vi "Actor Core.vi"(8 "error in":errorcluster, 11 "Nested in":refnum<class "Top Level.lvclass">) -> (0 "error out":errorcluster, 3 "Actor out":refnum<class "Actor.lvclass">)   [LabVIEW 2021, in "Top Level.lvlib" / "Top Level.lvclass"]
doc: "(<B>Filename</B>: Actor Framework.lvlib:Actor.lvclass:Actor Core.vi)\n\nReceives messages to the actor, reacts to them, and initiates any error handling that may shut the actor down.\n\nDescendant classes may override this VI to append parallel tasks for the actor to complete while it handles messages. Overrides use the Call Parent Method node."
uses:
  Top Level.lvclass
  C:/Program Files/National Instruments/LabVIEW 2021/vi.lib/ActorFramework/Actor/Actor.lvclass
  <vilib>/ActorFramework/Actor/Actor.lvclass
  <vilib>/ActorFramework/Actor/Actor.lvclass/Actor.ctl
  <vilib>/ActorFramework/Message Enqueuer/Message Enqueuer.lvclass/Message Enqueuer.ctl
  Top Level.lvclass/Top Level.ctl
  Top Level Messages/Password Authentication Msg/Password Authentication Msg.lvclass/Password Authentication Msg.ctl
  <vilib>/ActorFramework/Message Enqueuer/Init from Existing Queue.vi
  <vilib>/ActorFramework/Message Enqueuer/Enqueue.vi
  Top Level Messages/Password Authentication Msg/Password Authentication Msg.lvclass
  C:/Program Files/National Instruments/LabVIEW 2021/vi.lib/ActorFramework/Message/Message.lvclass
  <vilib>/ActorFramework/Stop Msg/Stop Msg.lvclass
  Top Level Messages/Reset Graph Msg/Reset Graph Msg.lvclass
  <vilib>/ActorFramework/Message Priority Queue/Priority Enqueue.vi
  <vilib>/ActorFramework/Message Enqueuer/Message Enqueuer.lvclass
  <vilib>/MGI/Panel Manager/Panel Actor/Panel Actor/Panel Actor.lvclass
panel:
  in  "Reset Graph":bool
  out "String":string="PH316 IV Curve Lab\n\nInstructions:\n\nCheck the user manual for hardware assembly.\n\nTo curve fit data to analytical functions, first export the necessary X-axis and Y-axis data:\nClick any of the three legends -> Export -> Export Data To ..\n\nCheck python's scipy.optimize.curve_fit module for details fitting your objective function to the data, further extracting unknown parameters of interest.\n\nZoom in / out, pane around, scale regions of interest, or individually control axes limits. Reset Graph at any time.\n\n\n\n\nService mode hidden from those not yet worthy.."
  out "XY Graph":cluster{"X":dbl[], "Y":dbl[]}[](graph)
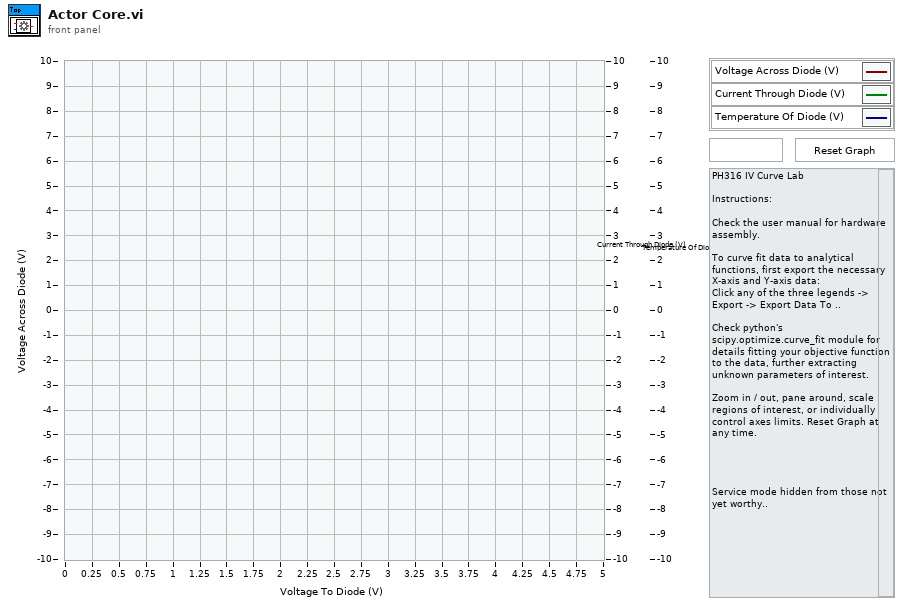
[diagram p1: front panel]
types:
  T1 = cluster{"Stop":refnum<user-event>, "XY Graph":refnum<user-event>}
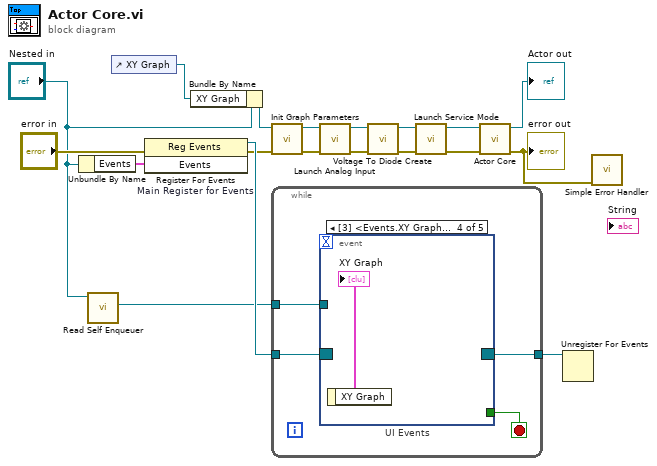
[diagram p0: block diagram]
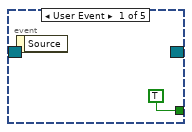
[diagram p2: hidden frame]
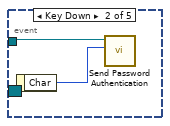
[diagram p3: hidden frame]
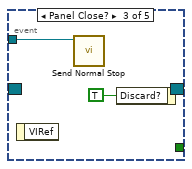
[diagram p4: hidden frame]
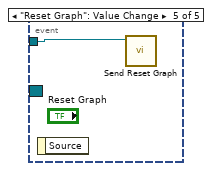
[diagram p5: hidden frame]
diagram:
  n1 = Unbundle By Name("Nested in") -> ("Events"=w17:T1)
  n2 = call <vilib>:"Read Self Enqueuer.vi"("Actor"="Nested in") -> ("Self Enqueuer"=w15:refnum<class "Message Enqueuer.lvclass">)  [unwired: 10 in]
  n3 = control-ref of="XY Graph"() -> (w1:refnum<vi>)
  n4 = register-events "Main Register for Events"(error in="error in", w17) -> (reference out=w18:refnum<event-registration>, error out=w5:errorcluster)  [unwired: 1 in]
  n5 = Bundle By Name(cluster="Nested in", "XY Graph"=w1) -> (w2:refnum<class "Top Level.lvclass">)
  n6 = call "Init Graph Parameters.vi"("error in (no error)"=w5, "Top Level in"=w2) -> ("error out"=w4:errorcluster, "Top Level out"=w3:refnum<class "Top Level.lvclass">)  [unwired: 8 in]
  n7 = while {
    tunnel: w18 -> [w23]
    tunnel: [w21] -> w16
    tunnel: w15 -> [w20]
    stop <- w22 stop-if-true
    n8 = event "UI Events" shown="[3] <Events.XY Graph>: User Event" {
      selector: w23 -> [_ _ _ _ _]
      dyn-events: [_ _ _ _ _] -> w21
      timeout: _ -> [_ _ _ _ _]
      tunnel: [TRUE _ _ _ _] -> w22
      tunnel: w20 -> [_ w26 w27 _ w30]
      event User Event {
        n9 = event-data() -> ()  [unwired: 1 in, 1 out]
      }
      event Key Down {
        n10 = event-data() -> ("Char"=w25:i16)  [unwired: 1 in]
        n11 = call "Send Password Authentication.vi"("Key"=w25, "Message Enqueuer"=w26) -> ()  [unwired: 8 in, 2 out]
      }
      event Panel Close? {
        n12 = event-data() -> ()  [unwired: 1 in, 1 out]
        n13 = call <vilib>:"Send Normal Stop.vi"("Message Enqueuer"=w27) -> ()  [unwired: 10 in, 1 out]
        n14 = event-data("Discard?"=TRUE) -> ()  [unwired: 1 in, 1 out]
      }
      event User Event {
        n15 = event-data() -> ("XY Graph"=→"XY Graph":cluster{"X":dbl[], "Y":dbl[]}[])  [unwired: 1 in]
      }
      event "Reset Graph": Value Change {
        n16 = event-data() -> ()  [unwired: 1 in, 1 out]
        n17 = call "Send Reset Graph.vi"("Message Enqueuer"=w30) -> ()  [unwired: 9 in, 2 out]
      }
    }
  }
  n18 = call "Launch Analog Input.vi"("error in (no error)"=w4, "Top Level in"=w3) -> ("error out"=w12:errorcluster, "Top Level out"=w13:refnum<class "Top Level.lvclass">)  [unwired: 8 in]
  n19 = call "Voltage To Diode Create.vi"("error in (no error)"=w12, "Top Level in"=w13) -> ("error out"=w10:errorcluster, "Top Level out"=w11:refnum<class "Top Level.lvclass">)  [unwired: 8 in]
  n20 = call "Launch Service Mode.vi"("error in (no error)"=w10, "Top Level in"=w11) -> ("error out"=w8:errorcluster, "Top Level out"=w9:refnum<class "Top Level.lvclass">)  [unwired: 8 in]
  n21 = call-parent "Actor Core.vi"("error in"=w8, "Panel Actor in"=w9) -> ("error out"=w7:errorcluster, "Actor out"=→"Actor out":refnum<class "Actor.lvclass">)  [unwired: 8 in]
  "error out" <- w7
  n22 = Unregister For Events(event registration refnum=w16) -> ()  [unwired: 1 in, 1 out]
  n23 = call <vilib>:"Simple Error Handler.vi"("error in (no error)"=w7) -> ()  [unwired: 4 in, 5 out]
